vi "BNC565 init Ch values.vi"(8 "error in (no error)":errorcluster, 10 "Settings":T2={"Delay"={"Ch 1"={"Value"=0.0, "Min"=0.0, "Max"=10.0, "StepSize"=1e-11, "Tolerance"=1e-11, "ValueActual"=0.0}, "Ch 2"={"Value"=0.0, "Min"=0.0, "Max"=10.0, "StepSize"=1e-11, "Tolerance"=1e-11, "ValueActual"=0.0}, "Ch 3"={"Value"=0.0, "Min"=0.0, "Max"=10.0, "StepSize"=1e-11, "Tolerance"=1e-11, "ValueActual"=0.0}, "Ch 4"={"Value"=0.0, "Min"=0.0, "Max"=10.0, "StepSize"=1e-11, "Tolerance"=1e-11, "ValueActual"=0.0}, "Ch 5"={"Value"=0.0, "Min"=0.0, "Max"=10.0, "StepSize"=1e-11, "Tolerance"=1e-11, "ValueActual"=0.0}, "Ch 6"={"Value"=0.0, "Min"=0.0, "Max"=10.0, "StepSize"=1e-11, "Tolerance"=1e-11, "ValueActual"=0.0}, "Ch 7"={"Value"=0.0, "Min"=0.0, "Max"=10.0, "StepSize"=1e-11, "Tolerance"=1e-11, "ValueActual"=0.0}, "Ch 8"={"Value"=0.0, "Min"=0.0, "Max"=10.0, "StepSize"=1e-11, "Tolerance"=1e-11, "ValueActual"=0.0}}, "VISA session"="COM1", "Save"=enum."off", "timeout"={"Value"=1.0, "Min"=0.0, "Max"=10.0, "StepSize"=1.0, "Tolerance"=0.0, "ValueActual"=0.0}, "Amplitude"={"Ch 1"={"Value"=5.0, "Min"=0.0, "Max"=12.0, "StepSize"=0.01, "Tolerance"=0.01, "ValueActual"=0.0}, "Ch 2"={"Value"=5.0, "Min"=0.0, "Max"=12.0, "StepSize"=0.01, "Tolerance"=0.01, "ValueActual"=0.0}, "Ch 3"={"Value"=5.0, "Min"=0.0, "Max"=12.0, "StepSize"=0.01, "Tolerance"=0.01, "ValueActual"=0.0}, "Ch 4"={"Value"=5.0, "Min"=0.0, "Max"=12.0, "StepSize"=0.01, "Tolerance"=0.01, "ValueActual"=0.0}, "Ch 5"={"Value"=5.0, "Min"=0.0, "Max"=12.0, "StepSize"=0.01, "Tolerance"=0.01, "ValueActual"=0.0}, "Ch 6"={"Value"=5.0, "Min"=0.0, "Max"=12.0, "StepSize"=0.01, "Tolerance"=0.01, "ValueActual"=0.0}, "Ch 7"={"Value"=5.0, "Min"=0.0, "Max"=12.0, "StepSize"=0.01, "Tolerance"=0.01, "ValueActual"=0.0}, "Ch 8"={"Value"=5.0, "Min"=0.0, "Max"=12.0, "StepSize"=0.01, "Tolerance"=0.01, "ValueActual"=0.0}}, "Width"={"Ch 1"={"Value"=1e-05, "Min"=0.0, "Max"=1.0, "StepSize"=1e-11, "Tolerance"=1e-11, "ValueActual"=0.0}, "Ch 2"={"Value"=1e-05, "Min"=0.0, "Max"=1.0, "StepSize"=1e-11, "Tolerance"=1e-11, "ValueActual"=0.0}, "Ch 3"={"Value"=1e-05, "Min"=0.0, "Max"=1.0, "StepSize"=1e-11, "Tolerance"=1e-11, "ValueActual"=0.0}, "Ch 4"={"Value"=1e-05, "Min"=0.0, "Max"=1.0, "StepSize"=1e-11, "Tolerance"=1e-11, "ValueActual"=0.0}, "Ch 5"={"Value"=1e-05, "Min"=0.0, "Max"=1.0, "StepSize"=1e-11, "Tolerance"=1e-11, "ValueActual"=0.0}, "Ch 6"={"Value"=1e-05, "Min"=0.0, "Max"=1.0, "StepSize"=1e-11, "Tolerance"=1e-11, "ValueActual"=0.0}, "Ch 7"={"Value"=1e-05, "Min"=0.0, "Max"=1.0, "StepSize"=1e-11, "Tolerance"=1e-11, "ValueActual"=0.0}, "Ch 8"={"Value"=1e-05, "Min"=0.0, "Max"=1.0, "StepSize"=1e-11, "Tolerance"=1e-11, "ValueActual"=0.0}}, "LocalSavingPath"=path "C:/temp", "Polarity"={"Ch 1"=enum."Positive", "Ch 2"=enum."Positive", "Ch 3"=enum."Positive", "Ch 4"=enum."Positive", "Ch 5"=enum."Positive", "Ch 6"=enum."Positive", "Ch 7"=enum."Positive", "Ch 8"=enum."Positive"}, "State"={"Ch 1"=enum."on", "Ch 2"=enum."on", "Ch 3"=enum."on", "Ch 4"=enum."on", "Ch 5"=enum."on", "Ch 6"=enum."on", "Ch 7"=enum."on", "Ch 8"=enum."on"}}, 11 "VISA Refnum in":refnum<visa-resource-name>) -> (0 "error out":errorcluster, 3 "VISA resource name out":refnum<visa-resource-name>)   [LabVIEW 2013, in "BNC565.lvclass"]
uses:
  BNC565.lvclass
  settingsBNC565_TypDef.ctl
  Device Drivers/shared/numericVariable_TypeDef.ctl
  OnOffTypeDef.ctl
  Channel Parameters.ctl
  Device Drivers/BaseDriver/BaseDriver.lvclass
panel:
  out "Array 2":T1[](array[typedef]) {"Chan Sync Source" items=["System (To)", "Channel A", "Channel B", "Channel C", "Channel D", "Channel E", "Channel F", "Channel G", "Channel H"]; "Chan Width" format="%.3p"; "Chan Delay" format="%.3p"; "Chan Lev Adjust" format="%.3p"; "Channel" items=["Channel A"=1, "Channel B"=2, "Channel C"=3, "Channel D"=4, "Channel E"=5, "Channel F"=6, "Channel G"=7, "Channel H"=8]}
  out "Array":T1[](array[typedef]) {"Chan Sync Source" items=["System (To)", "Channel A", "Channel B", "Channel C", "Channel D", "Channel E", "Channel F", "Channel G", "Channel H"]; "Chan Width" format="%.3p"; "Chan Delay" format="%.3p"; "Chan Lev Adjust" format="%.3p"; "Channel" items=["Channel A"=1, "Channel B"=2, "Channel C"=3, "Channel D"=4, "Channel E"=5, "Channel F"=6, "Channel G"=7, "Channel H"=8]}
  # "Input"
  # "Normal\nSingle\nBurst"
  # "Burst"
  # "Duty Cycle"
  # "Output"
  # "Input"
  # "Normal\nSingle\nBurst"
  # "Burst"
  # "Duty Cycle"
  # "Output"
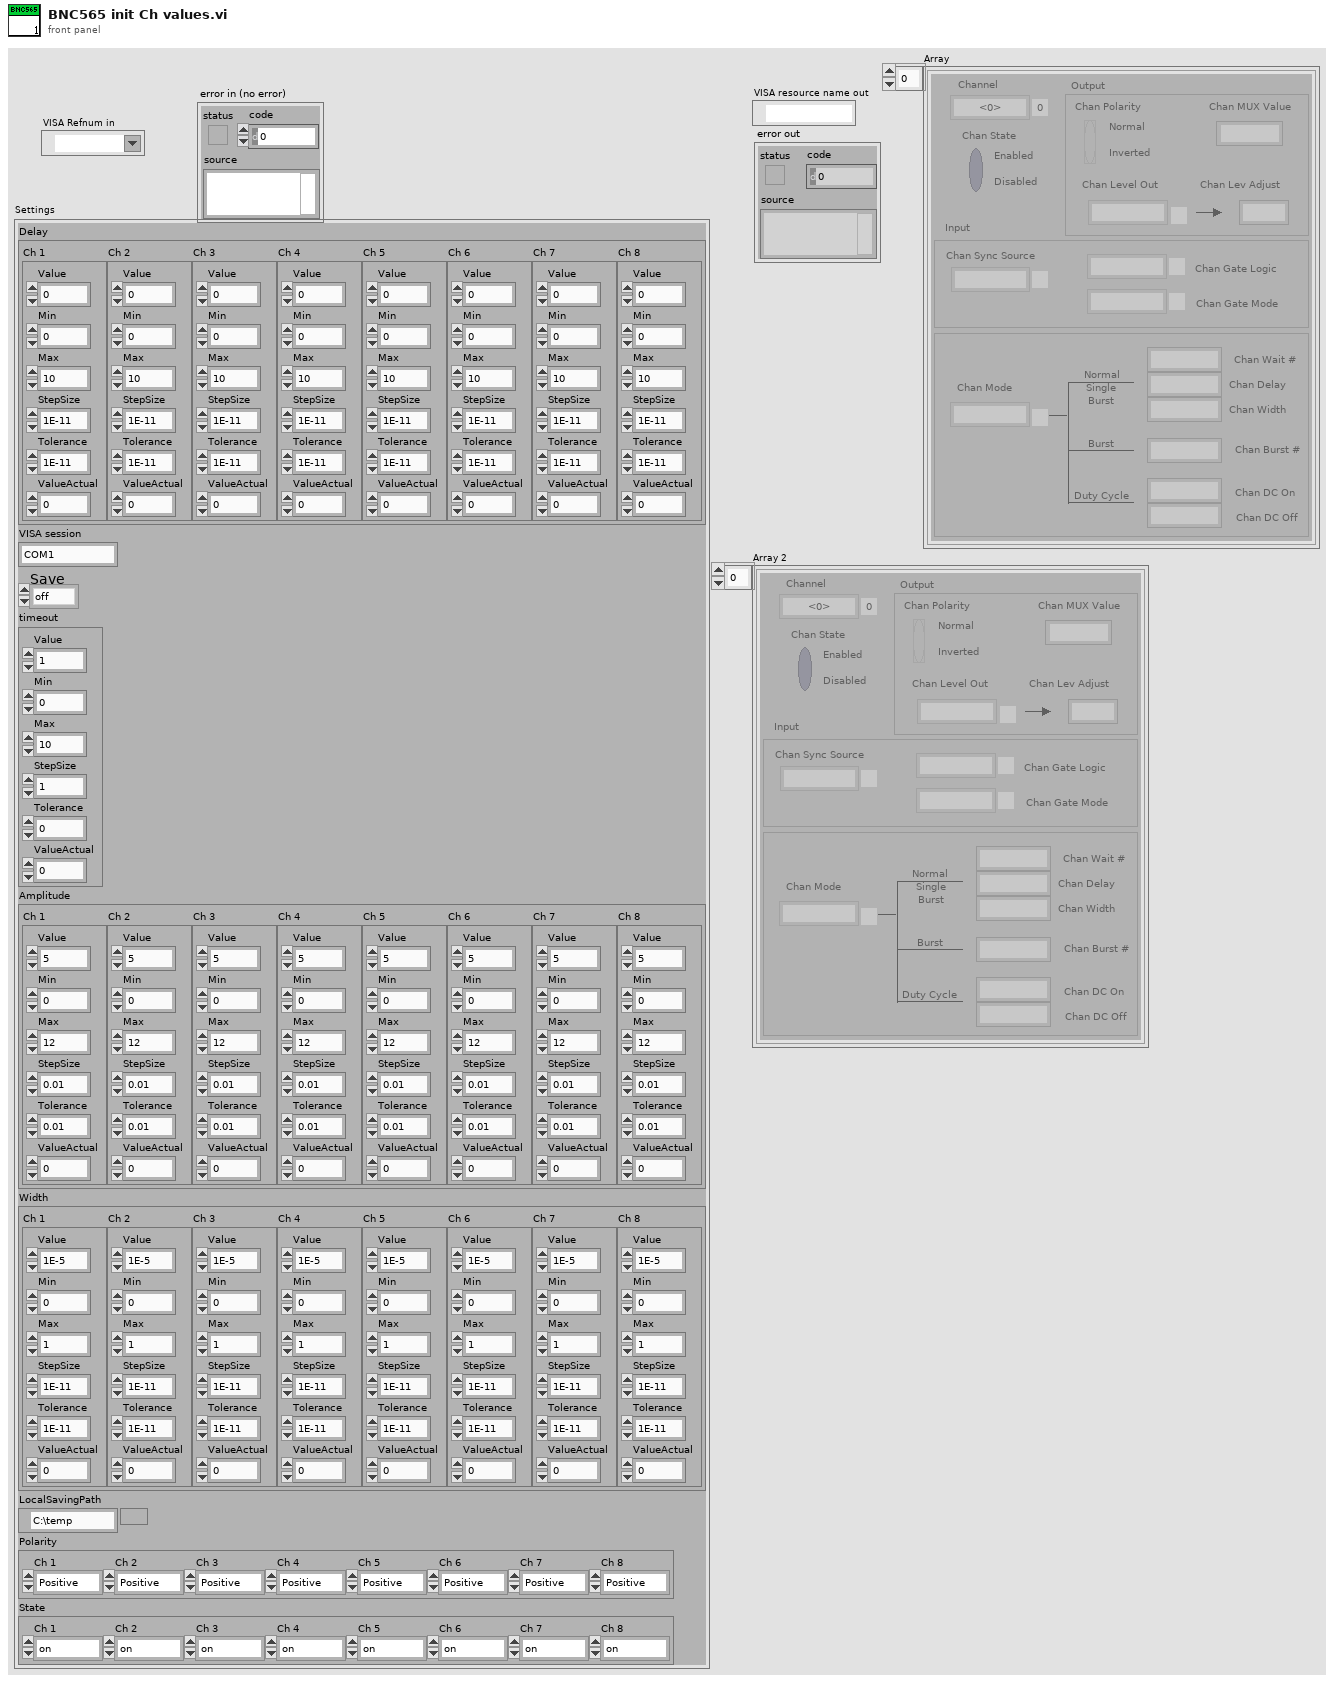
[diagram p1: front panel]
types:
  T1 = typedef "Channel Parameters.ctl" = cluster{"Channel":i32, "Chan State":bool, "Chan Sync Source":i32, "Chan Gate Logic":enum16{"Disabled", "Low", "High"}, "Chan Mode":enum16{"Normal", "Single", "Burst", "Duty Cycle"}, "Chan Wait #":i32, "Chan Delay":dbl, "Chan Width":dbl, "Chan Burst #":i32, "Chan DC On":i32, "Chan DC Off":i32, "Chan Polarity":bool, "Chan MUX Value":i32, "Chan Level Out":enum16{"TTL", "Adjustable", "35 Volt", "Optical"}, "Chan Lev Adjust":dbl, "Chan Gate Mode":enum16{"Disabled", "Pulse Inhibit", "Output Inhibit"}}
  T2 = typedef "BNC565.lvclass/settingsBNC565_TypDef.ctl" = cluster{"Delay":cluster{"Ch 1":T3, "Ch 2":T3, "Ch 3":T3, "Ch 4":T3, "Ch 5":T3, "Ch 6":T3, "Ch 7":T3, "Ch 8":T3}, "VISA session":string, "Save":T4, "timeout":T3, "Amplitude":cluster{"Ch 1":T3, "Ch 2":T3, "Ch 3":T3, "Ch 4":T3, "Ch 5":T3, "Ch 6":T3, "Ch 7":T3, "Ch 8":T3}, "Width":cluster{"Ch 1":T3, "Ch 2":T3, "Ch 3":T3, "Ch 4":T3, "Ch 5":T3, "Ch 6":T3, "Ch 7":T3, "Ch 8":T3}, "LocalSavingPath":path, "Polarity":cluster{"Ch 1":enum16{"Positive", "Negative"}, "Ch 2":enum16{"Positive", "Negative"}, "Ch 3":enum16{"Positive", "Negative"}, "Ch 4":enum16{"Positive", "Negative"}, "Ch 5":enum16{"Positive", "Negative"}, "Ch 6":enum16{"Positive", "Negative"}, "Ch 7":enum16{"Positive", "Negative"}, "Ch 8":enum16{"Positive", "Negative"}}, "State":cluster{"Ch 1":enum16{"on", "off"}, "Ch 2":enum16{"on", "off"}, "Ch 3":enum16{"on", "off"}, "Ch 4":enum16{"on", "off"}, "Ch 5":enum16{"on", "off"}, "Ch 6":enum16{"on", "off"}, "Ch 7":enum16{"on", "off"}, "Ch 8":enum16{"on", "off"}}}
  T3 = typedef "BaseDriver.lvclass/numericVariable_TypeDef.ctl" = cluster{"Value":dbl, "Min":dbl, "Max":dbl, "StepSize":dbl, "Tolerance":dbl, "ValueActual":dbl}
  T4 = typedef "OnOffTypeDef.ctl" = enum16{"off", "on"}
  T5 = cluster{"Ch 1":T3, "Ch 2":T3, "Ch 3":T3, "Ch 4":T3, "Ch 5":T3, "Ch 6":T3, "Ch 7":T3, "Ch 8":T3}
  T6 = cluster{"Ch 1":enum16{"Positive", "Negative"}, "Ch 2":enum16{"Positive", "Negative"}, "Ch 3":enum16{"Positive", "Negative"}, "Ch 4":enum16{"Positive", "Negative"}, "Ch 5":enum16{"Positive", "Negative"}, "Ch 6":enum16{"Positive", "Negative"}, "Ch 7":enum16{"Positive", "Negative"}, "Ch 8":enum16{"Positive", "Negative"}}
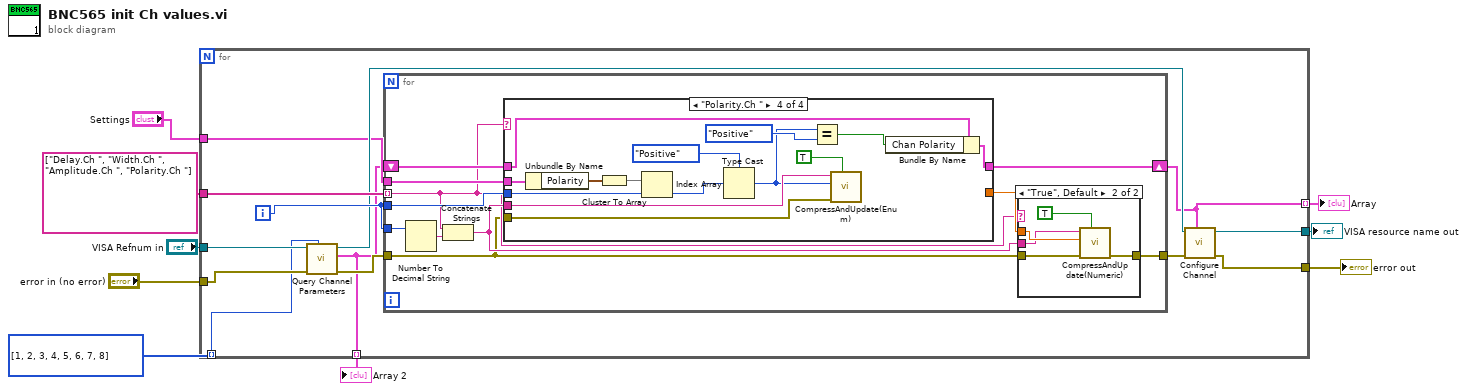
[diagram p0: block diagram]
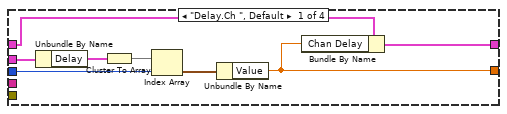
[diagram p3: hidden frame]
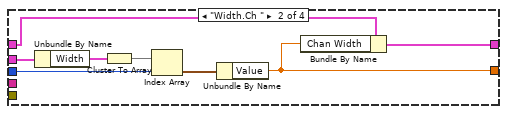
[diagram p4: hidden frame]
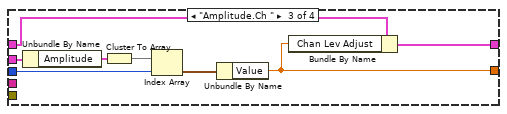
[diagram p5: hidden frame]
diagram:
  w1 = i32[] [1, 2, 3, 4, 5, 6, 7, 8] items=["Channel A"=1, "Channel B"=2, "Channel C"=3, "Channel D"=4, "Channel E"=5, "Channel F"=6, "Channel G"=7, "Channel H"=8]
  n1 = for {
    tunnel: string[] ["Delay.Ch ", "Width.Ch ", "Amplitude.Ch ", "Polarity.Ch "] -> [w22]
    tunnel: "Settings" -> [w16]
    tunnel: "VISA Refnum in" -> [w19]
    tunnel: [w15] -> w7
    tunnel: "error in (no error)" -> [w14]
    tunnel: [w13] -> w5
    tunnel: [w12] -> w3 mode=indexing
    tunnel: [w11] -> w2 mode=indexing
    tunnel: w1 -> [w10] mode=indexing
    i -> [w21]
    n2 = call "Query Channel Parameters.vi"("Channel (1:Chan A)"=w10, "error in (no error)"=w14, "VISA resource name"=w19) -> ("error out"=w18:errorcluster, "Chan Parameters"=w11:T1, "VISA resource name out"=w20:refnum<visa-resource-name>)  [unwired: 6 in]
    n3 = for {
      tunnel: w22 -> [w24] mode=indexing
      tunnel: w21 -> [w32]
      shift-right: [w30] -> w12
      shift-left: w11 -> [w31]
      tunnel: w16 -> [w29]
      tunnel: w21 -> [w28]
      tunnel: w18 -> [w23]
      tunnel: [w26] -> w17
      n4 = Number To Decimal String(number=w32) -> (decimal integer string=w33:string)  [unwired: 1 in]
      n5 = Concatenate Strings(w24, w33) -> (w25:string)
      n6 = case shown="\"Polarity.Ch \"" w24 {
        tunnel: w31 -> [w47 w55 w63 w77]
        tunnel: [w46 w54 w62 w76] -> w30
        tunnel: w29 -> [w45 w53 w61 w75]
        tunnel: w28 -> [w41 w49 w57 w72]
        tunnel: [w40 w48 w56 _] -> w27
        tunnel: w25 -> [_ _ _ w69]
        tunnel: w23 -> [_ _ _ w64]
        frame "Delay.Ch ", Default {
          n7 = Unbundle By Name(w45) -> ("Delay"=w44:T5)
          n8 = Cluster To Array(cluster=w44) -> (array=w43:T3[])
          n9 = Index Array(array=w43, index=w41) -> (element=w42:T3)
          n10 = Unbundle By Name(w42) -> ("Value"=w40:dbl)
          n11 = Bundle By Name(cluster=w47, "Chan Delay"=w40) -> (w46:T1)
        }
        frame "Width.Ch " {
          n12 = Unbundle By Name(w53) -> ("Width"=w52:T5)
          n13 = Cluster To Array(cluster=w52) -> (array=w51:T3[])
          n14 = Index Array(array=w51, index=w49) -> (element=w50:T3)
          n15 = Unbundle By Name(w50) -> ("Value"=w48:dbl)
          n16 = Bundle By Name(cluster=w55, "Chan Width"=w48) -> (w54:T1)
        }
        frame "Amplitude.Ch " {
          n17 = Unbundle By Name(w61) -> ("Amplitude"=w60:T5)
          n18 = Cluster To Array(cluster=w60) -> (array=w59:T3[])
          n19 = Index Array(array=w59, index=w57) -> (element=w58:T3)
          n20 = Unbundle By Name(w58) -> ("Value"=w56:dbl)
          n21 = Bundle By Name(cluster=w63, "Chan Lev Adjust"=w56) -> (w62:T1)
        }
        frame "Polarity.Ch " {
          n22 = Unbundle By Name(w75) -> ("Polarity"=w74:T6)
          n23 = Cluster To Array(cluster=w74) -> (array=w73:enum16{"Positive", "Negative"}[])
          n24 = Index Array(array=w73, index=w72) -> (element=w68:enum16{"Positive", "Negative"})
          n25 = Type Cast(type=enum16{"Positive", "Negative"}."Positive" ("Polarity.Ch 1"), x=w68) -> (*(type *) &x=w66:enum16{"Positive", "Negative"})
          n26 = Equal?(x=w66, y=enum16{"Positive", "Negative"}."Positive" ("trigger slope")) -> (x = y?=w65:bool)
          n27 = call "CompressAndUpdate(Enum).vi"("force CVT update (false)"=TRUE, "error in"=w64, "enum variant"=w66, "command or variable name"=w69) -> ()  [unwired: 7 in, 1 out]
          n28 = Bundle By Name(cluster=w77, "Chan Polarity"=w65) -> (w76:T1)
        }
      }
      n29 = case shown="\"True\", Default" w24 {
        tunnel: w27 -> [_ w39]
        tunnel: w23 -> [w34 w37]
        tunnel: [w34 w36] -> w26
        tunnel: w25 -> [_ w35]
        frame "Polarity.Ch " {
        }
        frame "True", Default {
          n30 = call "CompressAndUpdate(Numeric).vi"("force CVT update (false)"=TRUE, "error in"=w37, "Numeric"=w39, "command or variable name"=w35) -> ("error out"=w36:errorcluster)  [unwired: 7 in]
        }
      }
    }
    n31 = call "Configure Channel.vi"("Chan Parameters"=w12, "error in (no error)"=w17, "VISA resource name"=w20) -> ("error out"=w13:errorcluster, "VISA resource name out"=w15:refnum<visa-resource-name>)  [unwired: 7 in]
  }
  "VISA resource name out" <- w7
  "error out" <- w5
  "Array" <- w3
  "Array 2" <- w2
